vi "read_params.vi"(8 "error in (no error)":errorcluster, 11 "LogisticRegressionCV in":refnum<class "LogisticRegressionCV.lvclass">) -> (0 "error out":errorcluster, 2 "params":T1={"Cs"={"Cs_type"="int", "Cs_int"=10.0, "Cs_list"=[]}, "fit_intercept"=TRUE, "cv"=5.0, "dual"=FALSE, "penalty"="l2", "scoring"="None", "solver"="lbfgs", "tol"=0.0001, "max_iter"=100.0, "class_weight"={"class_weight_type"="None", "class_weight_dict"="{1:1.2,2:0.8,3:1.0}"}, "n_jobs"=1.0, "verbose"=0.0, "refit"=TRUE, "intercept_scaling"=1.0, "multi_class"="auto", "random_state"=0.0, "l1_ratios"={"l1_ratios_type"="None", "l1_ratios_list"=[]}}, 3 "LogisticRegressionCV out":refnum<class "LogisticRegressionCV.lvclass">)   [LabVIEW 2020, in "LogisticRegressionCV.lvclass"]
uses:
  LogisticRegressionCV.lvclass
  Controls/logistic_regression_cv_params.ctl
  LogisticRegressionCV.lvclass/LogisticRegressionCV.ctl
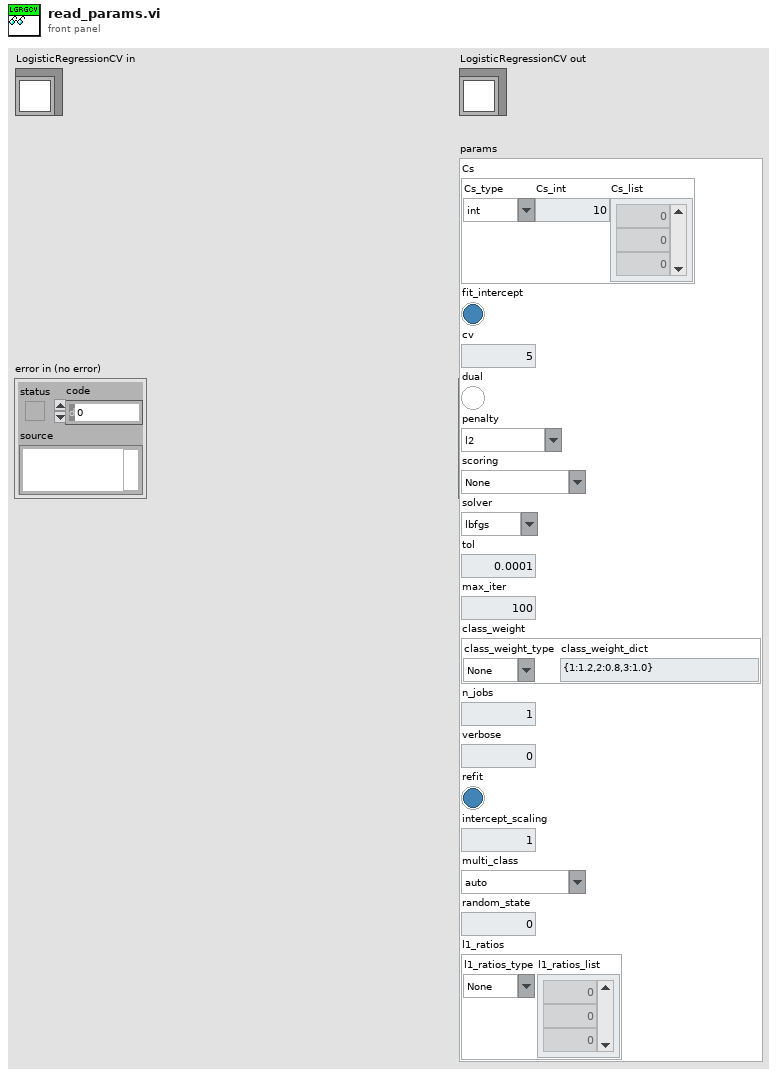
[diagram p1: front panel]
types:
  T1 = typedef "logistic_regression_cv_params.ctl" = cluster{"Cs":cluster{"Cs_type":string, "Cs_int":dbl, "Cs_list":dbl[]}, "fit_intercept":bool, "cv":dbl, "dual":bool, "penalty":string, "scoring":string, "solver":string, "tol":dbl, "max_iter":dbl, "class_weight":cluster{"class_weight_type":string, "class_weight_dict":string}, "n_jobs":dbl, "verbose":dbl, "refit":bool, "intercept_scaling":dbl, "multi_class":string, "random_state":dbl, "l1_ratios":cluster{"l1_ratios_type":string, "l1_ratios_list":dbl[]}}
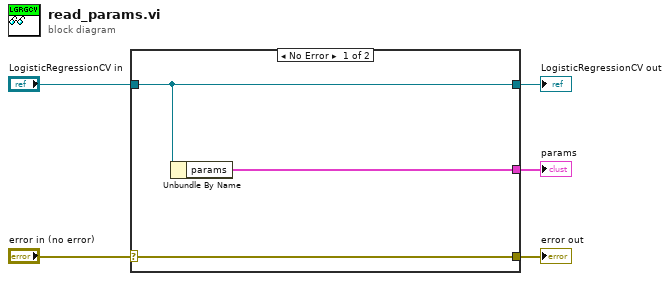
[diagram p0: block diagram]
diagram:
  n1 = case shown="No Error" "error in (no error)" {
    selector: "error in (no error)" -> [w8 w9]
    tunnel: [w8 w9] -> w4
    tunnel: [w7 w10] -> w2
    tunnel: "LogisticRegressionCV in" -> [w7 w10]
    tunnel: [w6 _] -> w1
    frame No Error {
      n2 = Unbundle By Name(w7) -> ("params"=w6:T1)
    }
    frame Error {
    }
  }
  "error out" <- w4
  "LogisticRegressionCV out" <- w2
  "params" <- w1
